vi "Teleop_Get_JoyStickValues.vi"() -> (1 "Joy0-POV":i32[](array[numeric]), 2 "Joy0-Buttons":bool[](array[boolean]), 3 "Joy0-Axes":dbl[](array[numeric]))   [LabVIEW 2019]
uses:
  Teleop_Globals.vi
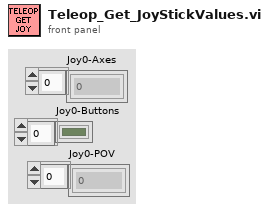
[diagram p1: front panel]
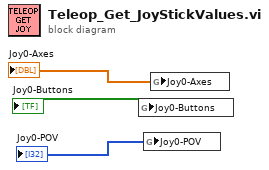
[diagram p0: block diagram]
diagram:
  n1 = global write "Teleop_Globals.vi" "Joy0-Buttons"("Joy0-Buttons") -> ()
  n2 = global write "Teleop_Globals.vi" "Joy0-POV"("Joy0-POV") -> ()
  n3 = global write "Teleop_Globals.vi" "Joy0-Axes"("Joy0-Axes") -> ()
